vi "main.vi"() -> ()   [LabVIEW 2018]
uses:
  Roda_Filtros/Roda_Filtros.lvclass
  Roda_Filtros/Roda_Filtros.lvclass/Roda_Filtros.ctl
panel:
  out "Current Filter":u16(ring)=1 items=["U"=1, "B"=2, "V"=3, "R"=4, "I"=5, "Clear"=6]
  in  "Serial Port":string="COM2"
  in  "Select Filter":u16(ring)=1 items=["U"=1, "B"=2, "V"=3, "R"=4, "I"=5, "Clear"=6]
  out "Error message":string
  in  "stop":bool
  out "communication status":bool
  # "Filter Wheel Control System (FWCS)"
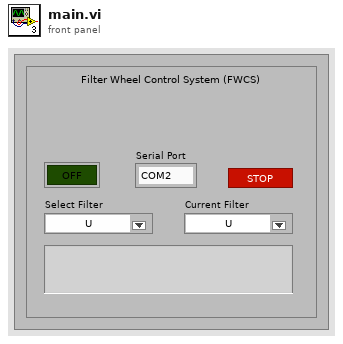
[diagram p1: front panel]
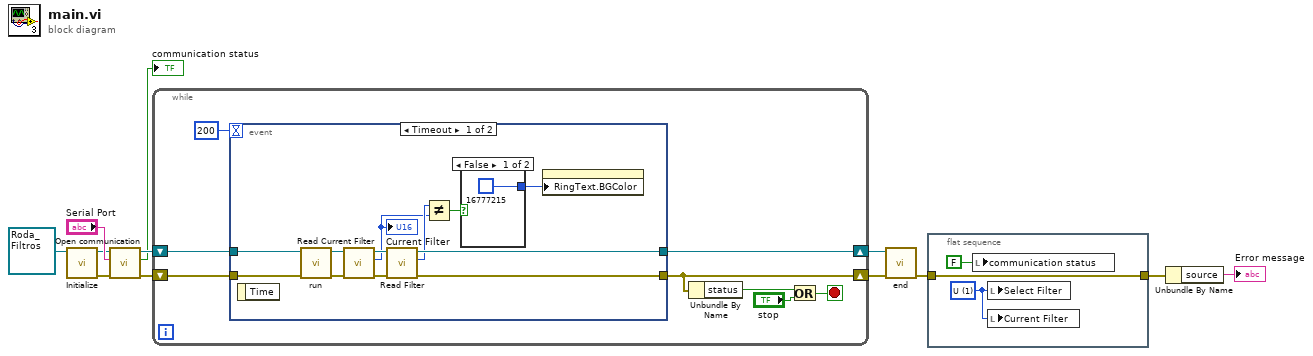
[diagram p0: block diagram]
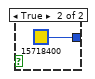
[diagram p2: hidden frame]
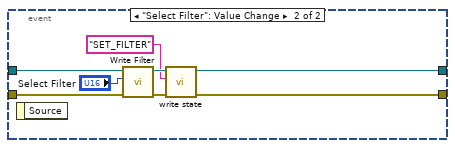
[diagram p3: hidden frame]
diagram:
  n1 = call "Initialize.vi"("Roda_Filtros in"=refnum<class "Roda_Filtros.lvclass"> refnum) -> ("error out"=w1:errorcluster, "Roda_Filtros out"=w2:refnum<class "Roda_Filtros.lvclass">)  [unwired: 9 in]
  n2 = call "Open communication.vi"("error in (no error)"=w1, "port"="Serial Port", "Roda_Filtros in"=w2) -> ("error out"=w10:errorcluster, "status"=→"communication status":bool, "Roda_Filtros out"=w11:refnum<class "Roda_Filtros.lvclass">)  [unwired: 6 in]
  n3 = while {
    shift-right: [w14] -> w4
    shift-left: w11 -> [w19]
    shift-right: [w18] -> w5
    shift-left: w10 -> [w20]
    stop <- w15 stop-if-true
    n4 = event shown="[0] Timeout" {
      selector: _ -> [_ _]
      dyn-events: _ -> [_ _]
      timeout: 200 -> [_ _]
      tunnel: w20 -> [w31 w41]
      tunnel: w19 -> [w32 w42]
      tunnel: [w26 w37] -> w18
      tunnel: [w25 w38] -> w14
      event Timeout {
        n5 = event-data() -> ()  [unwired: 1 in, 1 out]
        n6 = call "run.vi"("error in (no error)"=w31, "Roda_Filtros in"=w32) -> ("error out"=w30:errorcluster, "Roda_Filtros out"=w29:refnum<class "Roda_Filtros.lvclass">)  [unwired: 8 in]
        n7 = call "Read Current Filter.vi"("error in (no error)"=w30, "Roda_Filtros in"=w29) -> ("error out"=w27:errorcluster, "Current Filter"=w22:u16, "Roda_Filtros out"=w28:refnum<class "Roda_Filtros.lvclass">)  [unwired: 7 in]
        "Current Filter" <- w22
        n8 = call "Read Filter.vi"("error in (no error)"=w27, "Roda_Filtros in"=w28) -> ("error out"=w26:errorcluster, "Filter"=w23:u16, "Roda_Filtros out"=w25:refnum<class "Roda_Filtros.lvclass">)  [unwired: 7 in]
        n9 = Not Equal?(x=w23, y=w22) -> (x != y?=w24:bool)
        n10 = case shown="False" w24 {
          tunnel: [u32 16777215 u32 15718400] -> w21
          frame False {
          }
          frame True {
          }
        }
        n11 = property on="Current Filter" class="Ring (strict)"("RingText.BGColor"=w21) -> ()  [unwired: 2 in, 2 out]
      }
      event "Select Filter": Value Change {
        n12 = event-data() -> ()  [unwired: 1 in, 1 out]
        n13 = call "Write Filter.vi"("error in (no error)"=w41, "Filter"="Select Filter", "Roda_Filtros in"=w42) -> ("error out"=w36:errorcluster, "Roda_Filtros out"=w39:refnum<class "Roda_Filtros.lvclass">)  [unwired: 7 in]
        n14 = call "write state.vi"("error in (no error)"=w36, "State"="SET_FILTER", "Roda_Filtros in"=w39) -> ("error out"=w37:errorcluster, "Roda_Filtros out"=w38:refnum<class "Roda_Filtros.lvclass">)  [unwired: 7 in]
      }
    }
    n15 = Unbundle By Name(w18) -> ("status"=w17:bool)
    n16 = Or(x=w17, y="stop") -> (x .or. y?=w15:bool)
  }
  n17 = call "end.vi"("error in (no error)"=w5, "Roda_Filtros in"=w4) -> ("error out"=w6:errorcluster)  [unwired: 8 in, 1 out]
  n18 = flat-sequence {
    tunnel: w6 -> [w45]
    tunnel: [w45] -> w8
    frame #0 {
      w43 = u16 1 items=["U"=1, "B"=2, "V"=3, "R"=4, "I"=5, "Clear"=6] ("Select Filter")
      n19 = local write "communication status"(FALSE ("communication status")) -> ()
      n20 = local write "Select Filter"(w43) -> ()
      n21 = local write "Current Filter"(w43) -> ()
    }
  }
  n22 = Unbundle By Name(w8) -> ("source"=→"Error message":string)
